vi "complex derivative.vi"(6 "dt":dbl=10.0, 10 "omega":dbl[](array[numeric]), 11 "voltage":cdb[](array[numeric])) -> (3 "derivative":cdb[](array[numeric]))   [LabVIEW 2012]
uses:
  <vilib>/Analysis/NI_AALPro.lvlib
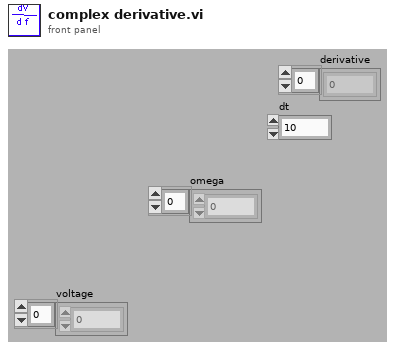
[diagram p1: front panel]
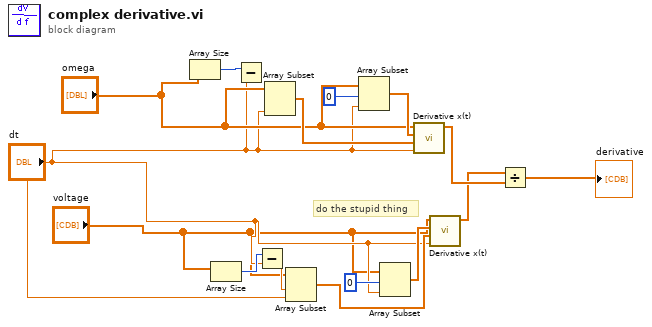
[diagram p0: block diagram]
diagram:
  # "do the stupid thing"
  n1 = Array Size(array="omega") -> (size(s)=w12:i32)
  n2 = Array Size(array="voltage") -> (size(s)=w9:i32)
  n3 = Subtract(x=w12, y="dt") -> ()  [unwired: 1 out]
  n4 = Subtract(x=w9, y="dt") -> (x-y=w8:dbl)
  n5 = Array Subset(array="omega", length="dt") -> (w13:dbl[])  [unwired: 1 in]
  n6 = Array Subset(array="voltage", index=w8, length="dt") -> (w6:cdb[])
  n7 = Array Subset(array="omega", index=0, length="dt") -> (w14:dbl[])
  n8 = Array Subset(array="voltage", index=0, length="dt") -> (w7:cdb[])
  n9 = call <vilib>:"Derivative x(t).vi"("dt"="dt", "Final Condition"=w13, "Initial Condition"=w14, "X"="omega") -> ("dX/dt"=w3:dbl[])  [unwired: 6 in, 1 out]
  n10 = call <vilib>:"Derivative x(t).vi"("dt"="dt", "Final Condition"=w6, "Initial Condition"=w7, "X"="voltage") -> ("dX/dt"=w2:dbl[])  [unwired: 6 in, 1 out]
  n11 = Divide(x=w2, y=w3) -> (x/y=→"derivative":dbl[])
